vi "Refresh Param Channels.vi"(8 "error in (no error)":errorcluster, 10 "Label":T1 {"scheduleBuildUnit" items=["Millisecond", "Microsecond"]}, 11 "Param Ref in":T5 format="%.0x") -> (0 "error out":errorcluster, 3 "Param Ref out":T5 format="%.0x")   [LabVIEW 2017, in "Ballard Arinc-429 System Explorer.lvlib"]
uses:
  Ballard Arinc-429 System Explorer.lvlib
  <vilib>/NI Veristand/Custom Device API/Custom Device Item Ref.ctl
  Controls/Ballard_Label.ctl
  Controls/Ballard_Word.ctl
  Controls/ARINCParam.ctl
  Shared/Controls and Global/TransferType.ctl
  <vilib>/NI Veristand/Custom Device API/Custom Device Channel Type.ctl
  Shared/Controls and Global/Global.vi
  <vilib>/NI Veristand/Custom Device API/Set Item Property (Variant).vi
  <vilib>/NI Veristand/Custom Device Tools/Custom Device Utility Library/NI VeriStand - Search for All Items by GUID.vi
  <vilib>/NI Veristand/Custom Device Tools/Custom Device Utility Library/NI VeriStand - Search for Item by GUID.vi
  Shared/Ballard Arinc-429 Shared.lvlib
  <vilib>/NI Veristand/Custom Device Tools/Custom Device Utility Library/Custom Device Utility Library.lvlib
  <vilib>/NI Veristand/Custom Device API/Custom Device API.lvlib
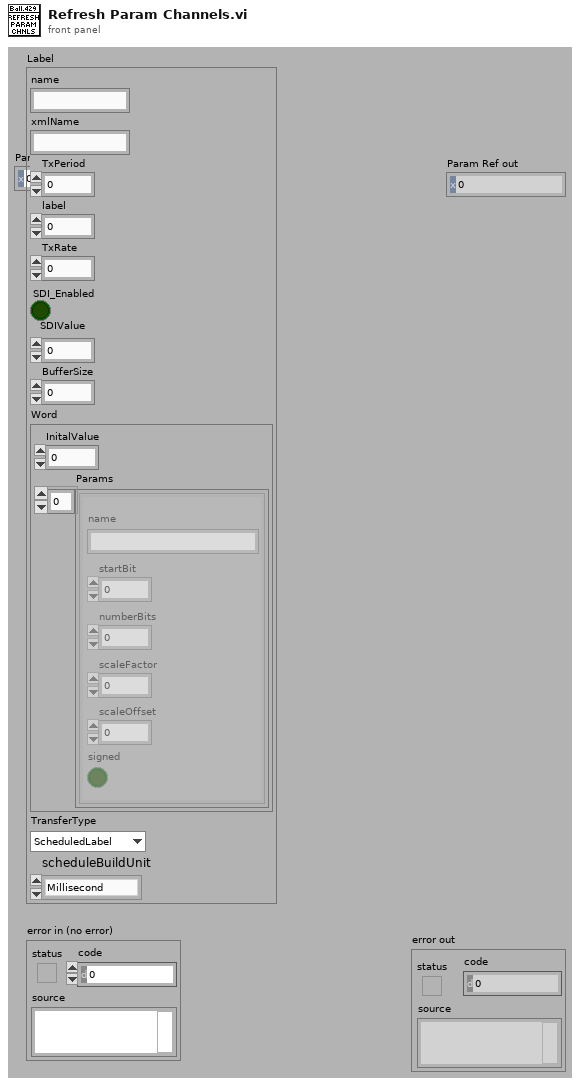
[diagram p1: front panel]
types:
  T1 = typedef "Ballard Arinc-429 System Explorer.lvlib/Ballard_Label.ctl" = cluster{"name":string, "xmlName":string, "TxPeriod":u32, "label":u32, "TxRate":dbl, "SDI_Enabled":bool, "SDIValue":u8, "BufferSize":u32, "Word":T2, "TransferType":T4, "scheduleBuildUnit":i32}
  T2 = typedef "Ballard Arinc-429 System Explorer.lvlib/Ballard_Word.ctl" = cluster{"InitalValue":u32, "Params":T3[]}
  T3 = typedef "Ballard Arinc-429 System Explorer.lvlib/ARINCParam.ctl" = cluster{"name":string, "startBit":i32, "numberBits":i32, "scaleFactor":dbl, "scaleOffset":dbl, "signed":bool}
  T4 = typedef "Ballard Arinc-429 Shared.lvlib/TransferType.ctl" = enum16{"ScheduledLabel", "Acyclic", "Block", "Strobe"}
  T5 = typedef "Custom Device API.lvlib/Custom Device Item Ref.ctl" = u64
  T6 = typedef "Custom Device API.lvlib/Custom Device Item Info.ctl" = cluster{"Name":string, "Is Channel":bool, "GUID":string, "Is Waveform":bool}
  T7 = typedef "Custom Device API.lvlib/Custom Device Channel Type.ctl" = enum16{"Input", "Output"}
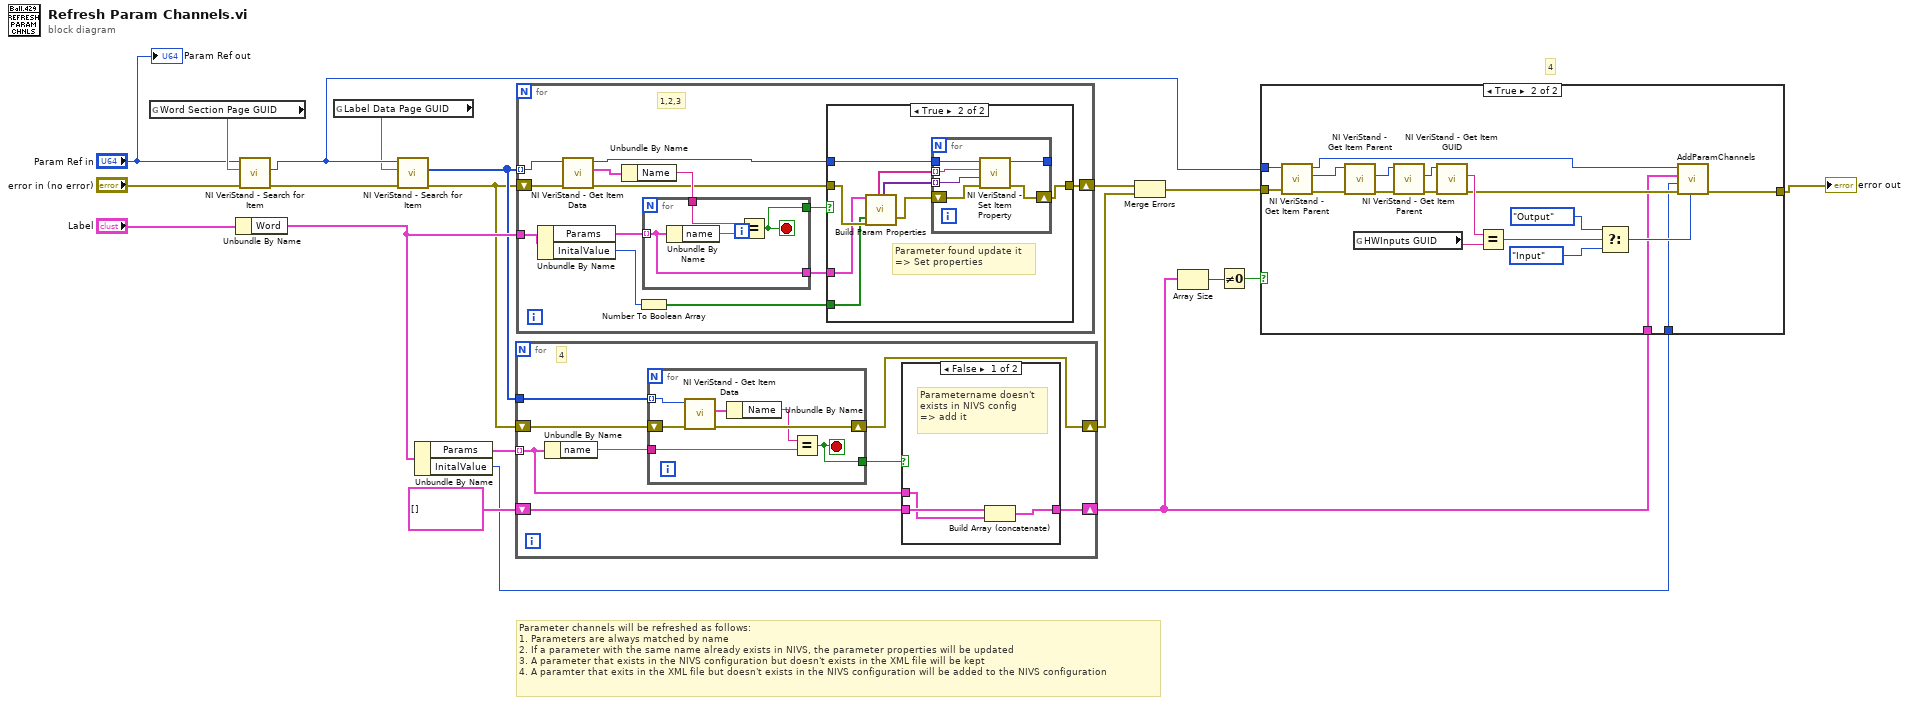
[diagram p0: block diagram]
diagram:
  # "4"
  # "Parameter channels will be refreshed as follows:\n1. Parameters are always matched by name\n2. If a parameter with the same name already exists in NIVS, the parameter properties will be updated\n3. A parameter that exists in the NIVS configuration but doesn't exists in the XML file will be kept\n4. A paramter that exits in the XML file but doesn't exists in the NIVS configuration will be added to the NIVS configuration"
  n1 = global read "Global.vi" "Word Section Page GUID"() -> (w18:string)
  n2 = Unbundle By Name("Label") -> ("Word"=w16:T2)
  n3 = call-poly <vilib>:"NI VeriStand - Search for Item.vi"("error in"="error in (no error)", "Item GUID"=w18, "Section Ref in"="Param Ref in") -> ("error out"=w14:errorcluster, "Item Ref"=w17:T5)  [unwired: 5 in, 2 out]
  n4 = global read "Global.vi" "Label Data Page GUID"() -> (w12:string)
  n5 = call-poly <vilib>:"NI VeriStand - Search for Item.vi"("error in"=w14, "Item GUID"=w12, "Section Ref in"=w17) -> ("error out"=w9:errorcluster, "Item Refs"=w10:T5[])  [unwired: 5 in, 2 out]
  n6 = Unbundle By Name(w16) -> ("Params"=w11:T3[], "InitalValue"=w1:u32)
  n7 = for {
    tunnel: w11 -> [w22] mode=indexing
    tunnel: w10 -> [w28]
    shift-right: [w23] -> w2
    shift-left: T3[] [] ("Params") -> [w24]
    shift-right: [w21] -> w7
    shift-left: w9 -> [w27]
    # "4"
    n8 = Unbundle By Name(w22) -> ("name"=w26:string)
    n9 = for {
      tunnel: w28 -> [w38] mode=indexing
      shift-right: [w36] -> w21
      shift-left: w27 -> [w39]
      tunnel: w26 -> [w35]
      tunnel: [w33] -> w25
      stop <- w33 stop-if-true
      n10 = call <vilib>:"NI VeriStand - Get Item Data.vi"("error in (no error)"=w39, "Item Ref in"=w38) -> ("error out"=w36:errorcluster, "Item Info"=w37:T6)  [unwired: 6 in, 2 out]
      n11 = Unbundle By Name(w37) -> ("Name"=w34:string)
      n12 = Equal?(x=w34, y=w35) -> (x = y?=w33:bool)
    }
    n13 = case shown="False" w25 {
      tunnel: w24 -> [w31 w32]
      tunnel: [w30 w32] -> w23
      tunnel: w22 -> [w29 _]
      frame False {
        # "Parametername doesn't\nexists in NIVS config\n=> add it"
        n14 = Build Array (concatenate)(w31, w29) -> (w30:T3[])
      }
      frame True {
        # "Parametername \nexists in both NIVS\nconfiguration and\nXML file\n=> Nothing to do"
      }
    }
  }
  n15 = for {
    shift-right: [w42] -> w6
    shift-left: w9 -> [w49]
    tunnel: w10 -> [w50] mode=indexing
    tunnel: w16 -> [w52]
    # "1,2,3"
    n16 = Unbundle By Name(w52) -> ("Params"=w51:T3[], "InitalValue"=w41:u32)
    n17 = call <vilib>:"NI VeriStand - Get Item Data.vi"("error in (no error)"=w49, "Item Ref in"=w50) -> ("error out"=w44:errorcluster, "Item Info"=w48:T6, "Item Ref out"=w45:T5)  [unwired: 6 in, 1 out]
    n18 = Unbundle By Name(w48) -> ("Name"=w47:string)
    n19 = Number To Boolean Array(number=w41) -> (Boolean array=w40:bool[])
    n20 = for {
      tunnel: w51 -> [w68] mode=indexing
      tunnel: w47 -> [w70]
      tunnel: [w69] -> w46
      tunnel: [w68] -> w43
      stop <- w69 stop-if-true
      n21 = Unbundle By Name(w68) -> ("name"=w71:string)
      n22 = Equal?(x=w70, y=w71) -> (x = y?=w69:bool)
    }
    n23 = case shown="True" w46 {
      tunnel: w45 -> [_ w58]
      tunnel: w44 -> [w53 w61]
      tunnel: w43 -> [_ w60]
      tunnel: [w53 w55] -> w42
      tunnel: w40 -> [_ w54]
      frame False {
        # "Parameter not in XML\nDo not change it"
      }
      frame True {
        # "Parameter found update it\n=> Set properties"
        n24 = call "Build Param Properties.vi"("ARINC Parameter"=w60, "Word"=w54, "error in (no error)"=w61) -> ("Prop Names"=w56:string[], "Prop Values"=w57:variant[], "error out"=w59:errorcluster)  [unwired: 8 in, 6 out]
        n25 = for {
          shift-right: [w66] -> w55
          shift-left: w59 -> [w67]
          tunnel: [w65] -> _
          tunnel: w58 -> [w64]
          tunnel: w57 -> [w63] mode=indexing
          tunnel: w56 -> [w62] mode=indexing
          n26 = call-poly <vilib>:"NI VeriStand - Set Item Property.vi"("error in (no error)"=w67, "Value"=w63, "Property Name"=w62, "Item Ref in"=w64) -> ("error out"=w66:errorcluster, "Item Ref out"=w65:T5)  [unwired: 5 in, 1 out]
        }
      }
    }
  }
  n27 = Merge Errors(w6, w7) -> (w3:errorcluster)
  n28 = Array Size(array=w2) -> (size(s)=w5:i32)
  n29 = Not Equal To 0?(x=w5) -> (x != 0?=w4:bool)
  n30 = case shown="True" w4 {
    tunnel: w3 -> [w72 w76]
    tunnel: w1 -> [_ w80]
    tunnel: w2 -> [_ w79]
    tunnel: [w72 w78] -> w19
    tunnel: w17 -> [_ w73]
    frame False {
    }
    frame True {
      n31 = call <vilib>:"NI VeriStand - Get Item Parent.vi"("error in (no error)"=w76, "Item Ref in"=w73) -> ("error out"=w77:errorcluster, "Parent Ref"=w75:T5, "Item Ref out"=w74:T5)  [unwired: 6 in, 1 out]
      n32 = call <vilib>:"NI VeriStand - Get Item Parent.vi"("error in (no error)"=w77, "Item Ref in"=w75) -> ("error out"=w83:errorcluster, "Parent Ref"=w86:T5)  [unwired: 6 in, 2 out]
      n33 = global read "Global.vi" "HWInputs GUID"() -> (w89:string)
      n34 = call <vilib>:"NI VeriStand - Get Item Parent.vi"("error in (no error)"=w83, "Item Ref in"=w86) -> ("error out"=w84:errorcluster, "Parent Ref"=w85:T5)  [unwired: 6 in, 2 out]
      n35 = call <vilib>:"NI VeriStand - Get Item GUID.vi"("error in (no error)"=w84, "Item Ref in"=w85) -> ("error out"=w82:errorcluster, "GUID"=w90:string)  [unwired: 7 in, 1 out]
      n36 = Equal?(x=w90, y=w89) -> (x = y?=w91:bool)
      n37 = Select(t=Custom_Device_Channel_Type."Output" ("Type"), s=w91, f=Custom_Device_Channel_Type."Input" ("Type")) -> (s? t:f=w81:T7)
      n38 = call "AddParamChannels.vi"("Type"=w81, "error in"=w82, "Initial Value"=w80, "Parameters to add"=w79, "Node Ref In"=w74) -> ("error out"=w78:errorcluster)  [unwired: 5 in, 1 out]
    }
  }
  "error out" <- w19
  "Param Ref out" <- "Param Ref in"
